vi "ProdaNG.TestValueResult.New.vi"(8 "error in (no error)":errorcluster, 10 "TestValueResult":T1, 11 "dbHandle":i32) -> (0 "error out":errorcluster, 2 "TestValueResult 2":T1, 3 "dbHandle":i32)   [LabVIEW 2016]
doc: "This function changes the process step result, which is defined by a ProcessStepResult structure. A process step result can either be set intentionally or leave the check of the test step results and the resulting changes to the DLL. In case, that the DLL changes the Process Result, the mdTime of the according Product is set to the current time and the mdProcessStepId is set to this process step. \nThe automatic check stands to the following rule:\n1. It is checked, if all test steps have the Status IO.\nIf the result of the test is IO, the status 1 (IO) is set in the test value result, otherwise the status 0 (NIO), respective 5 (IO Repeat) or 6 (NIO Repeat) in case of a repeat.\nParameter:\nhandle is an Integer, which is returned by the function Login() at the creation of a new connection.\nisRepeat shows, if this step is a repeat.\nprocessStepResult is a pointer on a ProcessStepResult structure, which elements must be prefilled. The structure must be defined and filled in the calling program. Changes can only be made on the elements StatusId, startTime and endTime. If the Endtime is not set, it is automatically filled with the current time by the DLL. \nThe element statusId is of particular importance:\nIf this element is passed with the value -1, the DLL makes a check on the test step results and sets the changeable elements automatically. Otherwise the returned values for status, start time and end time are set.\n\nReturncodes:\n0 No error\n< 0 ORACLE Error code\n6 (ERROR_INVALID_HANDLE) in case of an invalid handle\n1403 Record does not exist"
uses:
  Controls/ProdaNG.TestValueResult.ctl
  Controls/ProdaNG.TestValueResultSize.ctl
  prodllNG.dll
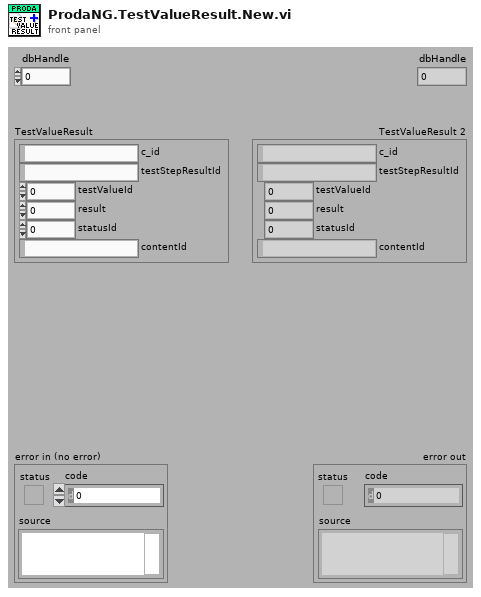
[diagram p1: front panel]
types:
  T1 = typedef "ProdaNG.TestValueResult.ctl" = cluster{"c_id":string, "testStepResultId":string, "testValueId":i32, "result":dbl, "statusId":i32, "contentId":string}
  T2 = typedef "ProdaNG.TestValueResultSize.ctl" = cluster{"c_id":i32, "testStepResultId":i32, "testValueId":i32, "result":i32, "statusId":i32, "contentId":i32}
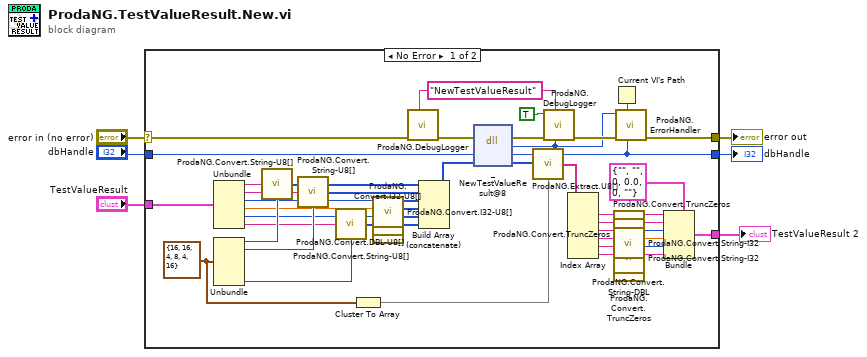
[diagram p0: block diagram]
diagram:
  n1 = case shown="No Error" "error in (no error)" {
    selector: "error in (no error)" -> [w34 w55]
    tunnel: [w31 w55] -> w5
    tunnel: [w30 w54] -> w4
    tunnel: "dbHandle" -> [w33 w54]
    tunnel: "TestValueResult" -> [w32 w53]
    tunnel: [w7 w53] -> w1
    frame No Error {
      w14 = T2 {"c_id"=16, "testStepResultId"=16, "testValueId"=4, "result"=8, "statusId"=4, "contentId"=16} ("TestValueResultSize")
      w49 = "NewTestValueResult" ("cmd")
      n2 = Unbundle(w32) -> ("c_id"=w51:string, "testStepResultId"=w52:string, "testValueId"=w39:i32, "result"=w38:dbl, "statusId"=w28:i32, "contentId"=w27:string)
      n3 = Unbundle(w14) -> ("c_id"=w43:i32, "testStepResultId"=w41:i32, "contentId"=w25:i32)  [unwired: 3 out]
      n4 = call "ProdaNG.Convert.String-U8[].vi"("Input String"=w51, "Size"=w43) -> ("Output"=w42:u8[])
      n5 = call "ProdaNG.Convert.String-U8[].vi"("Input String"=w52, "Size"=w41) -> ("Output"=w40:u8[])
      n6 = call "ProdaNG.Convert.String-U8[].vi"("Input String"=w27, "Size"=w25) -> ("Output"=w26:u8[])
      n7 = Cluster To Array(cluster=w14) -> (array=w13:i32[])
      n8 = call "ProdaNG.Convert.I32-U8[].vi"("32bit integer"=w39) -> ("unsigned byte array"=w37:u8[])  [unwired: 10 in]
      n9 = call "ProdaNG.Convert.DBL-U8[].vi"("dbl"=w38) -> ("unsigned byte array"=w36:u8[])  [unwired: 10 in]
      n10 = call "ProdaNG.Convert.I32-U8[].vi"("32bit integer"=w28) -> ("unsigned byte array"=w29:u8[])  [unwired: 10 in]
      n11 = call "ProdaNG.DebugLogger.vi"("cmd"=w49, "error in (no error)"=w34) -> ("error out"=w44:errorcluster)  [unwired: 9 in]
      n12 = Build Array (concatenate)(w42, w40, w37, w36, w29, w26) -> (w35:u8[])
      n13 = dll-call lib="D:/maszup/svn/LineTrace/trunk/SOFTWARE/sources/Database/ProdaNG/prodllNG.dll" fn="_NewTestValueResult@8" ("ProDll.dll:InitProDll")(error in=w44, "dbHandle"=w33, "testValueResult"=w35) -> (error out=w47:errorcluster, "return type"=w45:i32, "dbHandle"=w30:i32, "testValueResult"=w15:u8[])  [unwired: 2 in, 1 out]
      n14 = call "ProdaNG.Extract.U8[].vi"("unsigned byte array"=w15, "Sizes"=w13) -> ("Elements"=w17:string[])
      n15 = call "ProdaNG.DebugLogger.vi"("return type"=w45, "cmd"=w49, "error in (no error)"=w47, "done? (F)"=TRUE) -> ("error out"=w46:errorcluster)  [unwired: 7 in]
      n16 = Index Array(array=w17) -> (element #1=w19:string, element #2=w18:string, element #3=w24:string, element #4=w16:string, element #5=w10:string, element #6=w9:string)  [unwired: 6 in]
      n17 = Current VI's Path() -> (path=w50:path)
      n18 = call "ProdaNG.Convert.TruncZeros.vi"("string with \\0s"=w19) -> ("LV string"=w21:string)  [unwired: 10 in]
      n19 = call "ProdaNG.Convert.TruncZeros.vi"("string with \\0s"=w18) -> ("LV string"=w20:string)  [unwired: 10 in]
      n20 = call "ProdaNG.Convert.String-I32.vi"("unsigned byte string"=w24) -> ("32bit integer"=w23:i32)  [unwired: 10 in]
      n21 = call "ProdaNG.Convert.String-DBL.vi"("unsigned byte string"=w16) -> ("dbl integer"=w22:dbl)  [unwired: 10 in]
      n22 = call "ProdaNG.Convert.String-I32.vi"("unsigned byte string"=w10) -> ("32bit integer"=w11:i32)  [unwired: 10 in]
      n23 = call "ProdaNG.Convert.TruncZeros.vi"("string with \\0s"=w9) -> ("LV string"=w8:string)  [unwired: 10 in]
      n24 = call "ProdaNG.ErrorHandler.vi"("dbHandleIn"=w30, "Path"=w50, "error in"=w46, "output_parameter"=w45) -> ("error out"=w31:errorcluster)  [unwired: 7 in]
      n25 = Bundle(cluster=T1 {"c_id"="", "testStepResultId"="", "testValueId"=0, "result"=0.0, "statusId"=0, "contentId"=""} ("TestValueResult"), "c_id"=w21, "testStepResultId"=w20, "testValueId"=w23, "result"=w22, "statusId"=w11, "contentId"=w8) -> (w7:T1)
    }
    frame Error {
    }
  }
  "error out" <- w5
  "dbHandle" <- w4
  "TestValueResult 2" <- w1
